vi "RedMoRaceTiming_2020.vi"() -> ()   [LabVIEW 2018]
uses:
  <vilib>/event_ctls.llb/eventvkey.ctl
  <vilib>/Utility/miscctls.llb/LVRowAndColumnUnsignedTypeDef.ctl
  <vilib>/Utility/file.llb/Write Delimited Spreadsheet (string).vi
panel:
  out "Duplicate Bib #s":string[](array[string])
  in  "Clear Next Bib":bool
  out "File Path":path
  in  "SAVE TO FILE":bool
  in  "CLEAR ARRAYS":bool
  out "Total Control Times":i32
  out "ArrayOfControlTimeMarkers":string[](array[string])
  out "Finish Table":string[][](table)
  out "Total Bibs":i32
  out "Total Times":i32
  out "VKey":T1
  out "ArrayOfBibs":string[](array[string])
  out "*(type *) &x":string
  out "Char":i16
  out "ArrayOfTimes":string[](array[string])
  in  "Next Bib":string
  out "Time":string
  # "Bib"
  # "Time"
  # "CT?"
  # "Index"
  # "Instructions:\nSPACE BAR - log time only\nR key - log control time (bib + time)\nENTER (number pad) - log bib only starting from last control time or last bib"
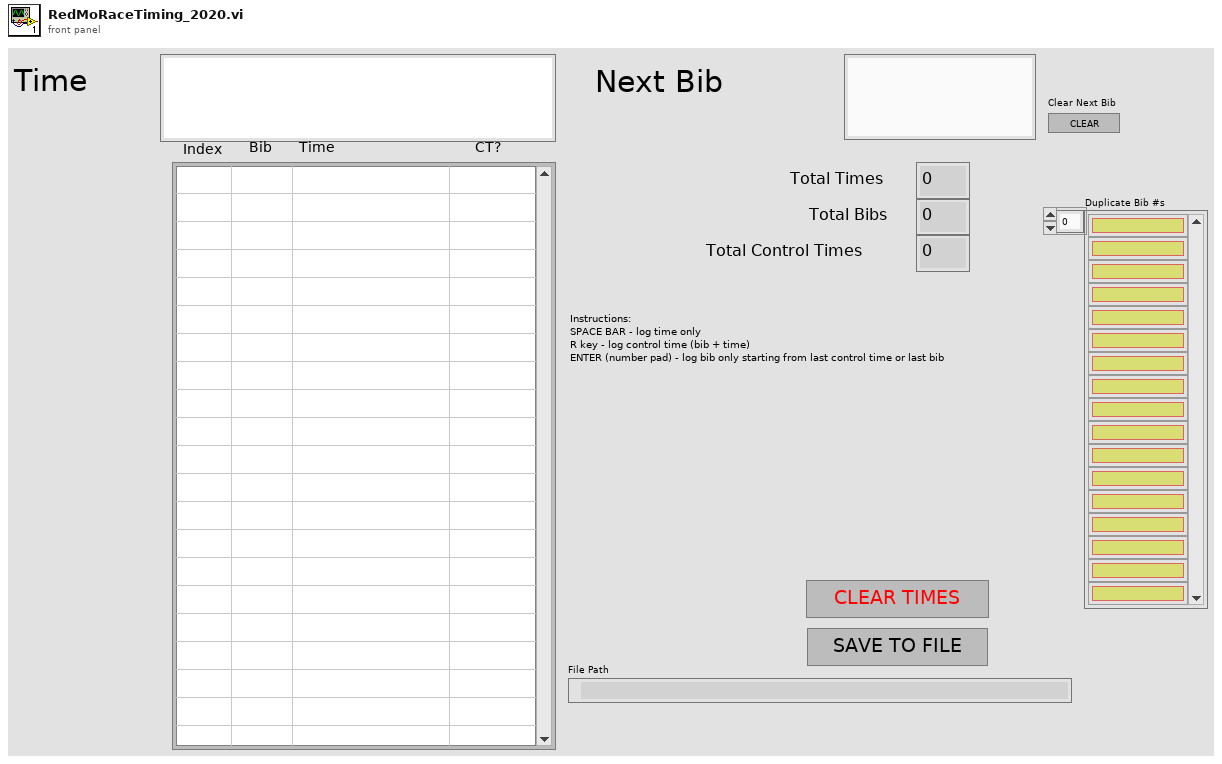
[diagram p1: front panel]
types:
  T1 = typedef "eventvkey.ctl" = enum16{"ASCII", "Enter", "Return", "Shift", "Ctrl", "Alt", "Cmd", "Opt", "Caps", "NumLock", "Clear", "Break", "Up", "Down", "Left", "Right", "Insert", "Delete", "Home", "End", "PageUp", "PageDown", "Escape", "Help", "Pause", "ScrollLock", "F1", "F2", "F3", "F4", "F5", "F6", "F7", "F8", "F9", "F10", "F11", "F12", "F13", "F14", "F15", "F16", "F17", "F18", "F19", "F20", "F21", "F22", "F23", "F24", "Play", "VolumeUp", "VolumeDown", "Mute", "Two Byte Char"}
  T2 = typedef "LVRowAndColumnUnsignedTypeDef.ctl" = cluster{"Row":u32, "Column":u32}
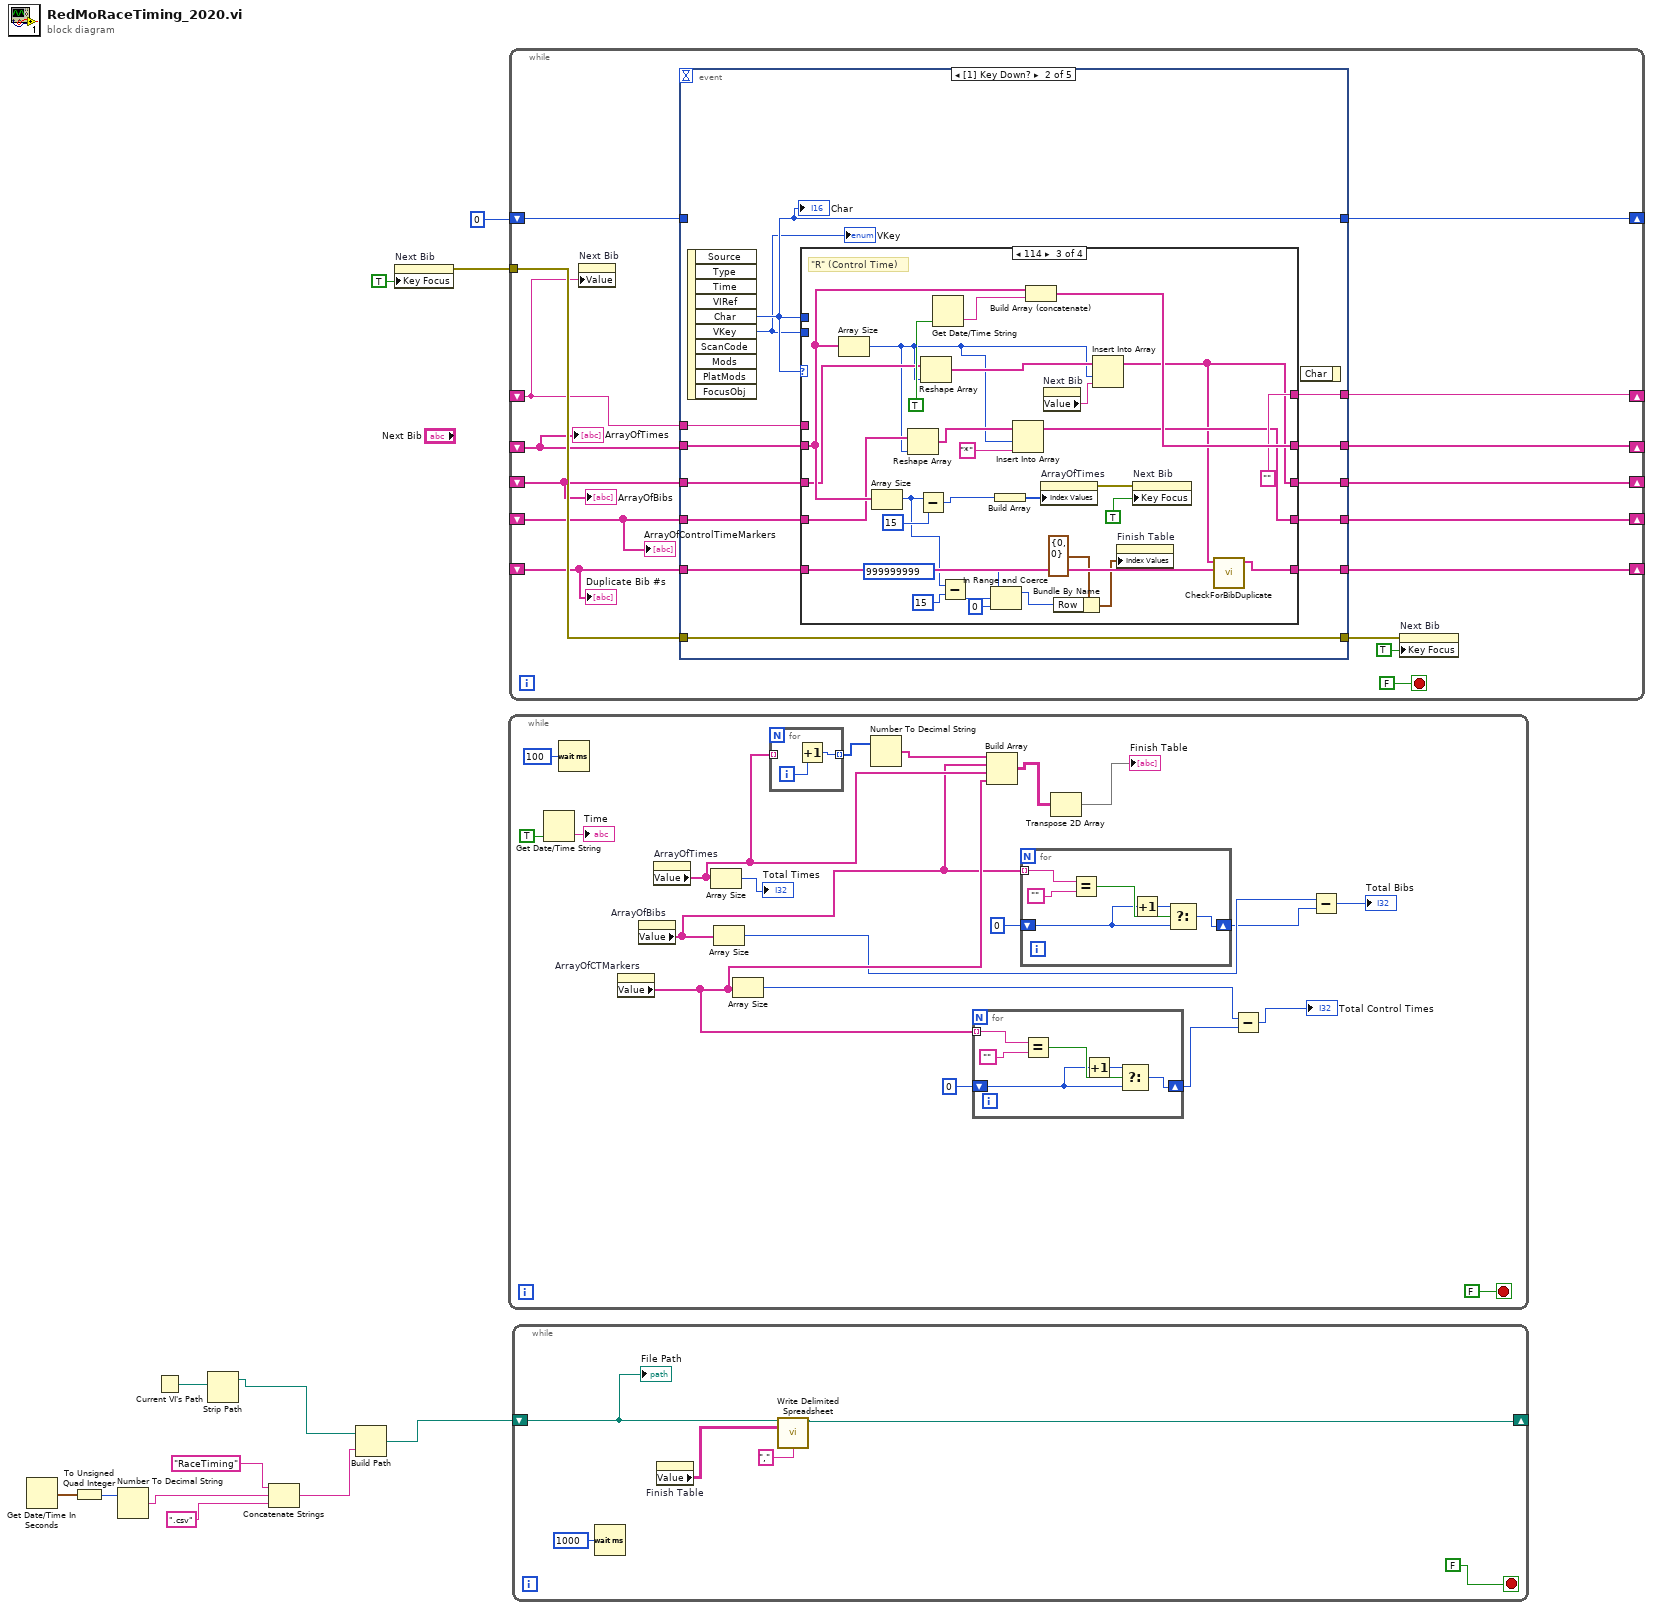
[diagram p0: block diagram]
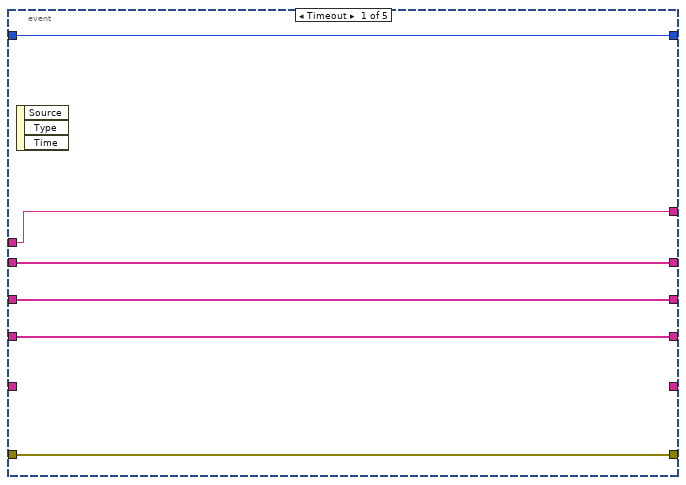
[diagram p2: hidden frame]
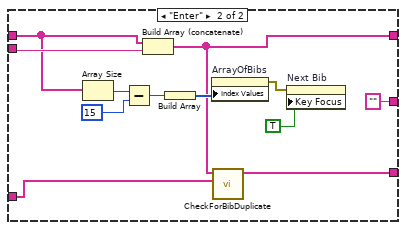
[diagram p4: hidden frame]
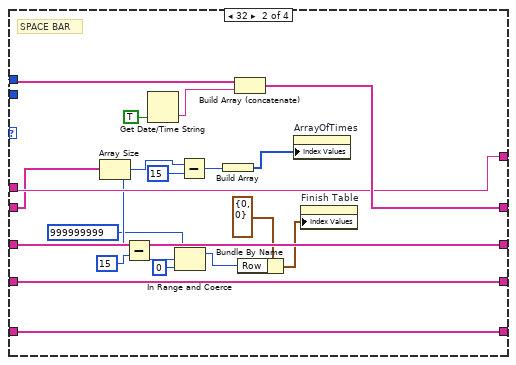
[diagram p5: hidden frame]
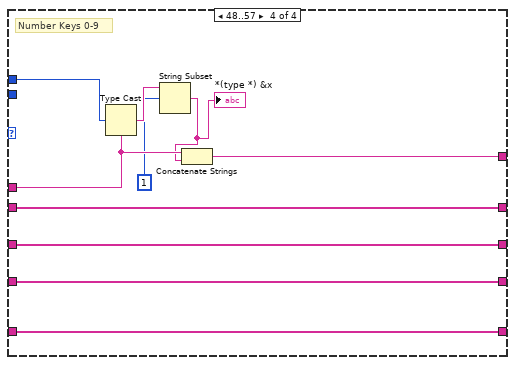
[diagram p6: hidden frame]
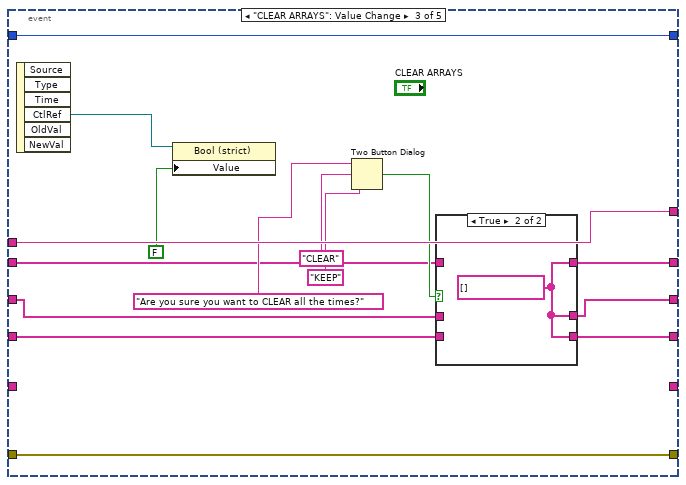
[diagram p7: hidden frame]
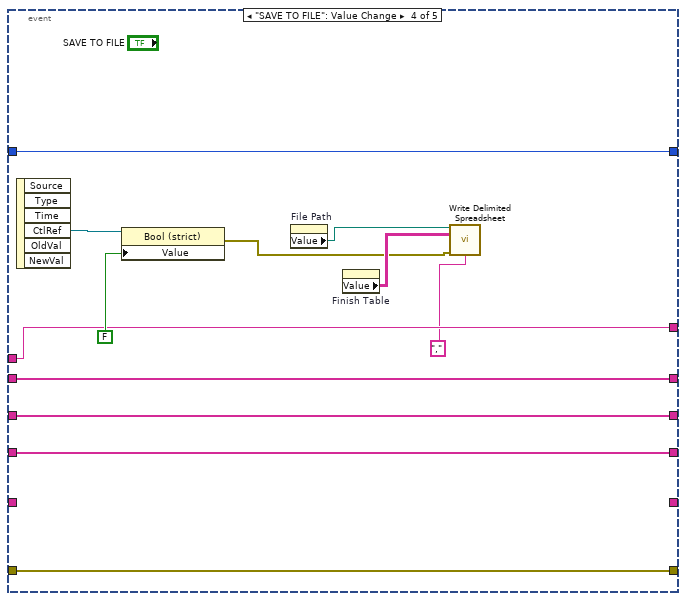
[diagram p9: hidden frame]
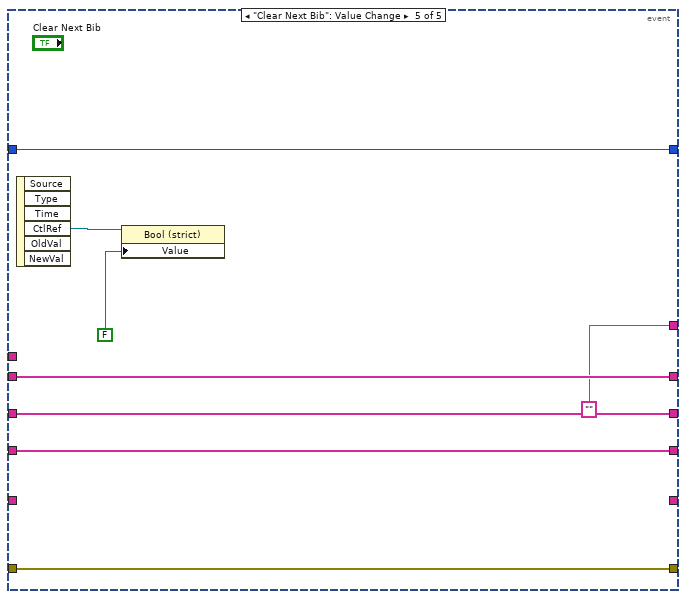
[diagram p10: hidden frame]
diagram:
  n1 = Get Date/Time In Seconds() -> (seconds since 1Jan1904=w4:timestamp)
  n2 = To Unsigned Quad Integer(1:w4) -> (0:w3:u64)
  n3 = Number To Decimal String(number=w3) -> (decimal integer string=w2:string)  [unwired: 1 in]
  n4 = Current VI's Path() -> (path=w6:path)
  n5 = Strip Path(path=w6) -> (stripped path=w5:path)  [unwired: 1 out]
  n6 = Concatenate Strings("RaceTiming", w2, ".csv") -> (w8:string)
  n7 = Build Path(base path=w5, name or relative path=w8) -> (appended path=w1:path)
  n8 = property on="Next Bib" class="Str"("Key Focus"=TRUE) -> (error out=w11:errorcluster)  [unwired: 2 in, 1 out]
  n9 = while {
    stop <- FALSE stop-if-true
    n10 = Get Date/Time String(want seconds? (F)=TRUE) -> (time string=→"Time":string)  [unwired: 2 in, 1 out]
    n11 = Wait (ms)(milliseconds to wait=u32 100) -> ()  [unwired: 1 out]
    n12 = property on="ArrayOfCTMarkers" class="Arr (strict)"() -> ("Value"=w26:string[])  [unwired: 2 in, 2 out]
    n13 = property on="ArrayOfBibs" class="Arr (strict)"() -> ("Value"=w13:string[])  [unwired: 2 in, 2 out]
    n14 = property on="ArrayOfTimes" class="Arr (strict)"() -> ("Value"=w16:string[])  [unwired: 2 in, 2 out]
    n15 = Array Size(array=w16) -> (size(s)=→"Total Times":i32)
    n16 = Array Size(array=w13) -> (size(s)=w20:i32)
    n17 = Array Size(array=w26) -> (size(s)=w24:i32)
    n18 = for {
      tunnel: w16 -> [_] mode=indexing
      tunnel: [w33] -> w15 mode=indexing
      i -> [w34]
      n19 = Increment(x=w34) -> (x+1=w33:i32)
    }
    n20 = Number To Decimal String(number=w15) -> (decimal integer string=w14:string[])  [unwired: 1 in]
    n21 = for {
      tunnel: w26 -> [w45] mode=indexing
      shift-right: [w43] -> w22
      shift-left: 0 -> [w41]
      n22 = Equal?(x=w45, y="") -> (x = y?=w44:bool)
      n23 = Increment(x=w41) -> (x+1=w42:i32)
      n24 = Select(t=w42, s=w44, f=w41) -> (s? t:f=w43:i32)
    }
    n25 = Build Array(w14, w13, w16, w26) -> (w29:string[][])
    n26 = for {
      tunnel: w13 -> [w39] mode=indexing
      shift-right: [w37] -> w19
      shift-left: 0 -> [w35]
      n27 = Equal?(x=w39, y="") -> (x = y?=w38:bool)
      n28 = Increment(x=w35) -> (x+1=w36:i32)
      n29 = Select(t=w36, s=w38, f=w35) -> (s? t:f=w37:i32)
    }
    n30 = Transpose 2D Array(2D array=w29) -> (transposed array=→"Finish Table":string[][])
    n31 = Subtract(x=w24, y=w22) -> (x-y=→"Total Control Times":i32)
    n32 = Subtract(x=w20, y=w19) -> (x-y=→"Total Bibs":i32)
  }
  n33 = while {
    shift-right: [w61] -> _
    shift-left: i16 0 ("Char") -> [w62]
    tunnel: w11 -> [w60]
    shift-right: [w59] -> _
    shift-left: _ -> [w58]
    shift-right: [w57] -> _
    shift-left: _ -> [w56]
    shift-right: [w54] -> _
    shift-left: _ -> [w55]
    shift-right: [w50] -> _
    shift-left: _ -> [w51]
    shift-right: [w47] -> _
    shift-left: _ -> [w48]
    stop <- FALSE stop-if-true
    n34 = property on="Next Bib" class="Str"("Value"=w56) -> ()  [unwired: 2 in, 2 out]
    n35 = event shown="[1] Key Down?" {
      selector: _ -> [_ _ _ _ _]
      dyn-events: _ -> [_ _ _ _ _]
      timeout: _ -> [_ _ _ _ _]
      tunnel: w62 -> [w68 _ w164 w188 w197]
      tunnel: [w68 w74 w164 w188 w197] -> w61
      tunnel: w60 -> [w67 w81 w177 w186 w196]
      tunnel: [w67 w81 w177 w186 w196] -> w52
      tunnel: w58 -> [w66 w80 w166 w190 w198]
      tunnel: [w66 w79 w165 w190 w198] -> w59
      tunnel: w56 -> [w63 w78 w178 w189 _]
      tunnel: [w63 w77 w178 w189 "" ("Bib Number")] -> w57
      tunnel: w55 -> [w64 w76 w168 w191 w199]
      tunnel: [w64 w75 w167 w191 w199] -> w54
      tunnel: w51 -> [w65 w72 w170 w192 w200]
      tunnel: [w65 w71 w171 w192 w200] -> w50
      tunnel: w48 -> [_ w70 _ _ _]
      tunnel: [_ w69 _ _ _] -> w47
      event Timeout {
        n36 = event-data() -> ()  [unwired: 1 in, 3 out]
      }
      event Key Down? {
        n37 = event-data() -> ("Char"=w74:i16, "VKey"=w73:T1)  [unwired: 1 in, 8 out]
        "Char" <- w74
        "VKey" <- w73
        n38 = case shown="114" w74 {
          tunnel: w80 -> [w90 w117 w147 w163]
          tunnel: [w90 w122 w151 w163] -> w79
          tunnel: w78 -> [w88 w121 _ w160]
          tunnel: w74 -> [_ _ _ w162]
          tunnel: [w85 w121 "" ("Bib Number") w161] -> w77
          tunnel: w76 -> [w87 w120 w144 w156]
          tunnel: [w86 w120 w133 w156] -> w75
          tunnel: w73 -> [w89 _ _ _]
          tunnel: w72 -> [w84 w116 w140 w155]
          tunnel: [w84 w116 w136 w155] -> w71
          tunnel: w70 -> [w83 w106 w135 w154]
          tunnel: [w82 w106 w134 w154] -> w69
          frame 0, Default {
            n39 = case shown="Default" w89 {
              tunnel: w87 -> [w93 w103]
              tunnel: w88 -> [w92 w105]
              tunnel: [w93 w95] -> w86
              tunnel: [w92 "" ("Bib Number")] -> w85
              tunnel: w83 -> [w91 w96]
              tunnel: [w91 w94] -> w82
              frame Default {
              }
              frame "Enter" {
                n40 = Array Size(array=w103) -> (size(s)=w102:i32)
                n41 = Subtract(x=w102, y=15) -> (x-y=w99:i32)
                n42 = Build Array (concatenate)(w103, w105) -> (w95:string[])
                n43 = Build Array(w99) -> (w100:i32[])
                n44 = property on="ArrayOfBibs" class="Arr (strict)"("Index Values"=w100) -> (error out=w97:errorcluster)  [unwired: 2 in, 1 out]
                n45 = call "CheckForBibDuplicate.vi"("ArrayOfDuplicateBibNumbers"=w96, "ArrayOfBibs"=w95) -> ("ArrayOfDuplicateBibNumbers"=w94:string[])  [unwired: 9 in]
                n46 = property on="Next Bib" class="Str"(error in=w97, "Key Focus"=TRUE) -> ()  [unwired: 1 in, 2 out]
              }
            }
          }
          frame 32 {
            # "SPACE BAR"
            n47 = Array Size(array=w117) -> (size(s)=w112:i32)
            n48 = Subtract(x=w112, y=15) -> (x-y=w110:i32)
            n49 = Get Date/Time String(want seconds? (F)=TRUE) -> (time string=w123:string)  [unwired: 2 in, 1 out]
            n50 = In Range and Coerce(upper limit=999999999, x=w110, lower limit=0) -> (coerced(x)=w108:i32)  [unwired: 1 out]
            n51 = Subtract(x=w112, y=15) -> (x-y=w118:i32)
            n52 = Build Array(w118) -> (w119:i32[])
            n53 = Build Array (concatenate)(w117, w123) -> (w122:string[])
            n54 = Bundle By Name(cluster=T2 {"Row"=0, "Column"=0} ("Index Values"), "Row"=w108) -> (w113:T2)
            n55 = property on="ArrayOfTimes" class="Arr (strict)"("Index Values"=w119) -> ()  [unwired: 2 in, 2 out]
            n56 = property on="Finish Table" class="Tbl (strict)"("Index Values"=w113) -> ()  [unwired: 2 in, 2 out]
          }
          frame 114 {
            # "\"R\" (Control Time)"
            n57 = Array Size(array=w147) -> (size(s)=w137:i32)
            n58 = Array Size(array=w147) -> (size(s)=w125:i32)
            n59 = Reshape Array(w140, w137) -> (w138:string[])
            n60 = Subtract(x=w125, y=15) -> (x-y=w149:i32)
            n61 = Reshape Array(w144, w137) -> (w143:string[])
            n62 = Get Date/Time String(want seconds? (F)=TRUE) -> (time string=w152:string)  [unwired: 2 in, 1 out]
            n63 = Subtract(x=w125, y=15) -> (x-y=w129:i32)
            n64 = In Range and Coerce(upper limit=999999999, x=w129, lower limit=0) -> (coerced(x)=w127:i32)  [unwired: 1 out]
            n65 = Build Array(w149) -> (w150:i32[])
            n66 = Insert Into Array(array=w138, index=w137, new element="*") -> (w136:string[])
            n67 = Build Array (concatenate)(w147, w152) -> (w151:string[])
            n68 = property on="ArrayOfTimes" class="Arr (strict)"("Index Values"=w150) -> (error out=w141:errorcluster)  [unwired: 2 in, 1 out]
            n69 = property on="Next Bib" class="Str"() -> ("Value"=w145:string)  [unwired: 2 in, 2 out]
            n70 = Bundle By Name(cluster=T2 {"Row"=0, "Column"=0} ("Index Values"), "Row"=w127) -> (w130:T2)
            n71 = Insert Into Array(array=w143, index=w137, new element=w145) -> (w133:string[])
            n72 = property on="Finish Table" class="Tbl (strict)"("Index Values"=w130) -> ()  [unwired: 2 in, 2 out]
            n73 = property on="Next Bib" class="Str"(error in=w141, "Key Focus"=TRUE) -> ()  [unwired: 1 in, 2 out]
            n74 = call "CheckForBibDuplicate.vi"("ArrayOfDuplicateBibNumbers"=w135, "ArrayOfBibs"=w133) -> ("ArrayOfDuplicateBibNumbers"=w134:string[])  [unwired: 9 in]
          }
          frame 48..57 {
            # "Number Keys 0-9"
            n75 = Type Cast(type=w160, x=w162) -> (*(type *) &x=w159:string)
            n76 = String Subset(string=w159, offset (0)=1) -> (substring=w157:string)  [unwired: 1 in]
            "*(type *) &x" <- w157
            n77 = Concatenate Strings(w160, w157) -> (w161:string)
          }
        }
        n78 = event-data() -> ()  [unwired: 2 in, 1 out]
      }
      event "CLEAR ARRAYS": Value Change {
        n79 = event-data() -> ("CtlRef"=w176:refnum<vi>)  [unwired: 1 in, 5 out]
        n80 = property class="Bool (strict)"(reference=w176, "Value"=FALSE) -> ()  [unwired: 1 in, 2 out]
        n81 = Two Button Dialog(message="Are you sure you want to CLEAR all the times?", 1:"KEEP" ("F button name (\"Cancel\")"), 2:"CLEAR" ("T button name (\"OK\")")) -> (T button?=w169:bool)
        n82 = case shown="True" w169 {
          tunnel: [w181 w182] -> w171
          tunnel: w170 -> [w181 _]
          tunnel: [w180 w182] -> w167
          tunnel: w168 -> [w180 _]
          tunnel: w166 -> [w179 _]
          tunnel: [w179 w182] -> w165
          frame False {
          }
          frame True {
            w182 = string[] [] ("ArrayOfTimes")
          }
        }
      }
      event "SAVE TO FILE": Value Change {
        n83 = event-data() -> ("CtlRef"=w194:refnum<vi>)  [unwired: 1 in, 5 out]
        n84 = property class="Bool (strict)"(reference=w194, "Value"=FALSE) -> (error out=w184:errorcluster)  [unwired: 1 in, 1 out]
        n85 = property on="File Path" class="Path"() -> ("Value"=w187:path)  [unwired: 2 in, 2 out]
        n86 = property on="Finish Table" class="Tbl (strict)"() -> ("Value"=w185:string[][])  [unwired: 2 in, 2 out]
        n87 = call-poly <vilib>:"Write Delimited Spreadsheet.vi"("file path (dialog if empty)"=w187, "2D data"=w185, "error in (no error)"=w184, "delimiter (\\t)"="," ("delimiter (\\t)")) -> ()  [unwired: 10 in, 2 out]
      }
      event "Clear Next Bib": Value Change {
        n88 = event-data() -> ("CtlRef"=w202:refnum<vi>)  [unwired: 1 in, 5 out]
        n89 = property class="Bool (strict)"(reference=w202, "Value"=FALSE) -> ()  [unwired: 1 in, 2 out]
      }
    }
    n90 = property on="Next Bib" class="Str"(error in=w52, "Key Focus"=TRUE) -> ()  [unwired: 1 in, 2 out]
    "ArrayOfTimes" <- w58
    "ArrayOfBibs" <- w55
    "ArrayOfControlTimeMarkers" <- w51
    "Duplicate Bib #s" <- w48
  }
  n91 = while {
    shift-right: [w205] -> _
    shift-left: w1 -> [w206]
    stop <- FALSE stop-if-true
    n92 = Wait (ms)(milliseconds to wait=u32 1000) -> ()  [unwired: 1 out]
    n93 = property on="Finish Table" class="Tbl (strict)"() -> ("Value"=w204:string[][])  [unwired: 2 in, 2 out]
    n94 = call-poly <vilib>:"Write Delimited Spreadsheet.vi"("file path (dialog if empty)"=w206, "2D data"=w204, "delimiter (\\t)"="," ("delimiter (\\t)")) -> ("new file path (Not A Path if cancelled)"=w205:path)  [unwired: 11 in, 1 out]
    "File Path" <- w206
  }
